vi "Get Alarm DVR.vi"(8 "error in (no error)":errorcluster, 11 "Timed Door in":refnum<class "Timed Door.lvclass">) -> (0 "error out":errorcluster, 2 "Alarm DVR":refnum<data-value>, 3 "Timed Door out":refnum<class "Timed Door.lvclass">)   [LabVIEW 2018, in "Timed Door.lvclass"]
uses:
  Timed Door.lvclass
  Alarm/Alarm.lvclass
  Timed Door.lvclass/Timed Door.ctl
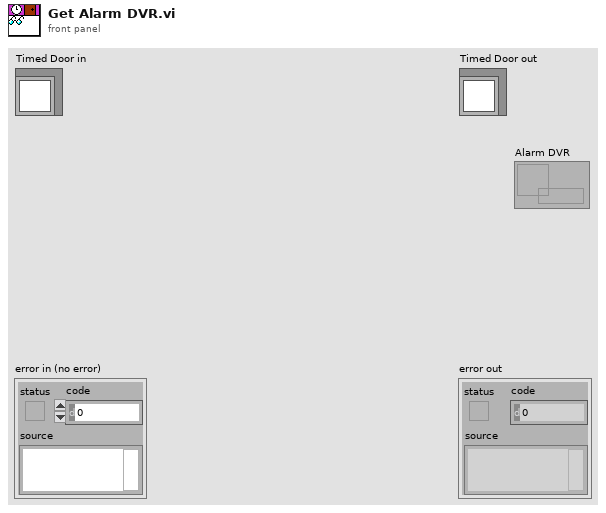
[diagram p1: front panel]
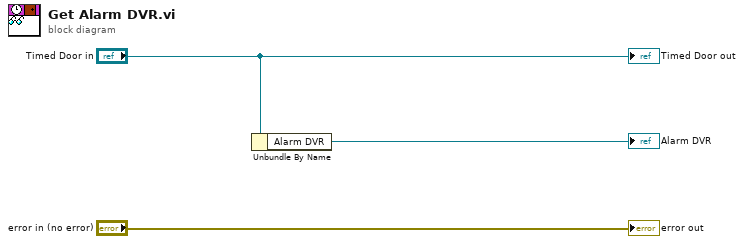
[diagram p0: block diagram]
diagram:
  n1 = Unbundle By Name("Timed Door in") -> ("Alarm DVR"=→"Alarm DVR":refnum<data-value>)
  "error out" <- "error in (no error)"
  "Timed Door out" <- "Timed Door in"
